vi "PKG_IMC_GetFunErrStrW.vi"() -> (3 "function return":u16)   [LabVIEW 2018, in "IMC_Pkg4xxx.lvlib"]
doc: "PKG_IMC_GetFunErrStrW();"
uses:
  IMC_Pkg4xxx.lvlib
  IMC_Pkg4xxx.dll
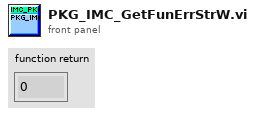
[diagram p1: front panel]
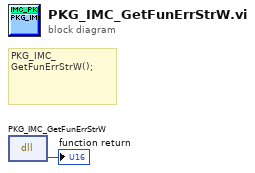
[diagram p0: block diagram]
diagram:
  # "PKG_IMC_GetFunErrStrW();"
  n1 = dll-call lib="PTH2\\abs D做的项目航天测量驱动电机IMCAppincLabview32\nIMC_Pkg4xxx.*" fn="PKG_IMC_GetFunErrStrW"() -> (→"function return":u16)  [unwired: 3 in, 2 out]
